vi "系统信息解析.vi"(11 "系统信息":u16[](array[numeric])) -> ()   [LabVIEW 2016, in "数据传输系统-06.lvlib"]
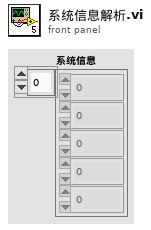
[diagram p1: front panel]
types:
  T1 = cluster{"CODMn固件信息":string, "氨氮固件信息":string, "总磷固件信息":string, "总氮固件信息":string, "CODCr固件信息":string}
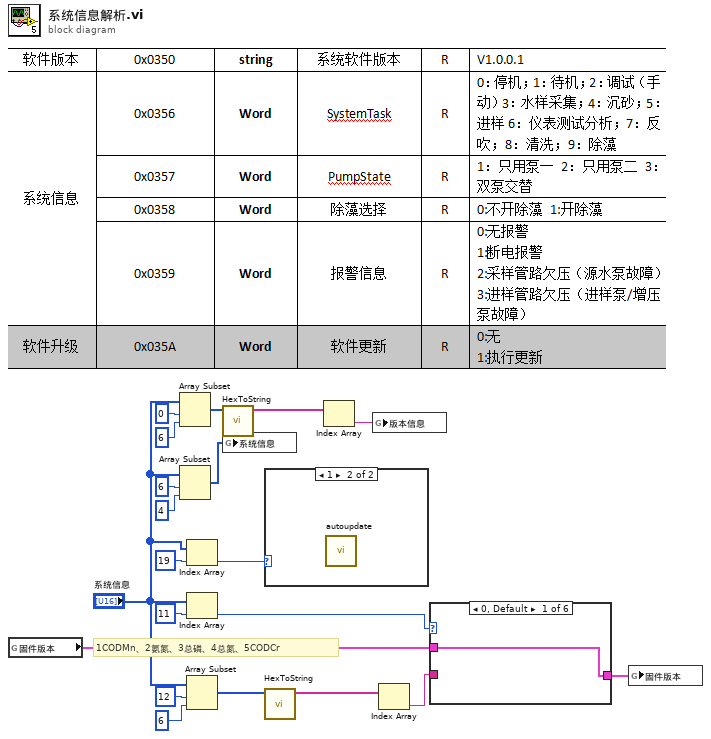
[diagram p0: block diagram]
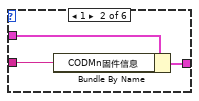
[diagram p3: hidden frame]
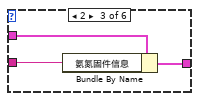
[diagram p4: hidden frame]
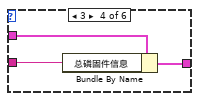
[diagram p5: hidden frame]
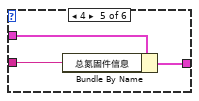
[diagram p6: hidden frame]
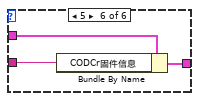
[diagram p7: hidden frame]
diagram:
  # "1CODMn、2氨氮、3总磷、4总氮、5CODCr"
  n1 = global read "全局1.vi" "固件版本"() -> (w7:T1)
  n2 = Array Subset(array="系统信息", index=0 ("索引"), length=6 ("长度")) -> (w16:u16[])
  n3 = Array Subset(array="系统信息", index=6 ("索引"), length=4 ("长度")) -> (w15:u16[])
  n4 = Index Array(array="系统信息", index=19 ("索引")) -> (element=w2:u16)
  n5 = Index Array(array="系统信息", index=11 ("索引")) -> (element=w5:u16)
  n6 = Array Subset(array="系统信息", index=12 ("索引"), length=6 ("长度")) -> (w8:u16[])
  n7 = call "HexToString.vi"("数组"=w16) -> ("STRING"=w14:string[])  [unwired: 10 in]
  n8 = global write "全局1.vi" "系统信息"(w15) -> ()
  n9 = case shown="1" w2 {
    frame 0, Default {
    }
    frame 1 {
      n10 = call "autoupdate.vi"() -> ()  [unwired: 12 in]
    }
  }
  n11 = call "HexToString.vi"("数组"=w8) -> ("STRING"=w10:string[])  [unwired: 10 in]
  n12 = Index Array(array=w14) -> (element=w13:string)  [unwired: 1 in]
  n13 = global write "全局1.vi" "版本信息"(w13) -> ()
  n14 = Index Array(array=w10) -> (element=w4:string)  [unwired: 1 in]
  n15 = case shown="0, Default" w5 {
    tunnel: w7 -> [w21 w24 w27 w30 w33 w36]
    tunnel: [w21 w23 w26 w29 w32 w35] -> w6
    tunnel: w4 -> [_ w22 w25 w28 w31 w34]
    frame 0, Default {
    }
    frame 1 {
      n16 = Bundle By Name(cluster=w24, "CODMn固件信息"=w22) -> (w23:T1)
    }
    frame 2 {
      n17 = Bundle By Name(cluster=w27, "氨氮固件信息"=w25) -> (w26:T1)
    }
    frame 3 {
      n18 = Bundle By Name(cluster=w30, "总磷固件信息"=w28) -> (w29:T1)
    }
    frame 4 {
      n19 = Bundle By Name(cluster=w33, "总氮固件信息"=w31) -> (w32:T1)
    }
    frame 5 {
      n20 = Bundle By Name(cluster=w36, "CODCr固件信息"=w34) -> (w35:T1)
    }
  }
  n21 = global write "全局1.vi" "固件版本"(w6) -> ()
